vi "FPGA Digitize and Protect.vi"() -> ()   [LabVIEW 2020]
doc: "Author: Scott Hannahs <sth@magnet.fsu.edu>\nCopyright 2018 Florida State University, All rights reserved."
uses:
  SCH Test Controls/SCH Fudge Factor Array.ctl
  SCH Test Controls/SCH Fudge Factor.ctl
  SCH Test Controls/SCH Layer Error Array.ctl
  SCH Data Controls/SCH Data 2 RT.ctl
  SCH Scaling Controls/SCH Scale Factor Array.ctl
  SCH Scaling Controls/SCH Scale Factor.ctl
  SCH Data Controls/SCH Layer Voltage Array.ctl
  Init Coil Calibration/FPGA Magnet Config.ctl
  SCH Scaling Controls/SCH Joint Scale Factor Array.ctl
  SCH Scaling Controls/SCH Joint Scale Factor.ctl
  SCH Test Controls/SCH CoWound Geometric Factor.ctl
  SCH Scaling Controls/SCH CoWound Scale Factor.ctl
  SCH Data Controls/SCH Joint Voltage Array.ctl
  SCH Data Controls/SCH CoWound Volt Array.ctl
  SCH Scaling Controls/SCH SC Bus Scale Factor Array.ctl
  SCH Scaling Controls/SCH SC Bus Scale Factor.ctl
  SCH Data Controls/SCH SC Bus Volt Array.ctl
  SCH Data Controls/SCH Data 2 RT Array.ctl
  SCH Data Controls/SCH Resistive Data Array.ctl
  SCH Data Controls/SCH FXP Type.ctl
  SCH Test Controls/SCH CoWound Volt Limit.ctl
  SCH Data Controls/SCH Raw Int Data.ctl
  SCH Scaling Controls/SCH Dump Resistor Scale Factor.ctl
  SCH Data Controls/SCH Pressure Array.ctl
  SCH Data Controls/Digitizer State Enum.ctl
  SCH Data Controls/SCH Int Data with Pressure.ctl
  <vilib>/rvi/Emulation/niFpgaGetClockAttributes.vi
  <vilib>/rvi/Emulation/niFpgaSctlEmulationGetInTimedLoop.vi
  <vilib>/rvi/Emulation/niFpgaEmulationReportErrorSimple.vi
  <vilib>/rvi/Emulation/niFpgaProcessEmulError.vi
  <vilib>/rvi/eio/common/nirviEmuTemplateMethod_errors.vi
  <vilib>/rvi/Emulation/niFpgaCriticalErrorInLSC.vi
  <vilib>/rvi/Emulation/niFpgaEmulationIsFPGAContextNoSignature.vi
  <vilib>/rvi/errors/niFpgaSetErrorForExecOnDevCompSimple.vi
  <vilib>/rvi/eio/common/nirviEmuReportErrorAndStop.vi
  <vilib>/rvi/DataTransferAndStorage/Container/Common/niFpgaContainerGetUniqueNameForEmu.vi
  <vilib>/rvi/FIFO/Fifo_Resource/nirvififoEmulationSetSize.vi
  <vilib>/rvi/FIFO/Fifo_Resource/nirviFifoEmulationQueueMgr.vi
  <instcachedir>/0/nirviFifoEmulationQueueMgr_E5CAEC123FF24DC58D834DCA3CDAA9B5.lvgen/nirviFifoEmulationQueueMgr_E5CAEC123FF24DC58D834DCA3CDAA9B5_006.vi
  <vilib>/Utility/error.llb/Clear Errors.vi
  <vilib>/rvi/FIFO/Fifo_Resource/nirvififoEmulationCreateLock.vi
  <vilib>/rvi/FIFO/Fifo_Resource/nirvififoEmulationObtainLock.vi
  <vilib>/rvi/FIFO/Fifo_Resource/nirvififoEmulationReleaseLock.vi
  <vilib>/rvi/occurrence/nirviWaitOnOccurrenceBase.vi
  <vilib>/rvi/errors/nirviReportUnexpectedCaseInternalError.vi
  <vilib>/rvi/errors/nirviReportUnexpectedCaseInternalError (U32).vi
  <instcachedir>/0/nirviFifoEmulationQueueMgr_E5CAEC123FF24DC58D834DCA3CDAA9B5.lvgen/nirviFifoEmulationQueueMgr_E5CAEC123FF24DC58D834DCA3CDAA9B5_010.vi
  <vilib>/rvi/FIFO/Fifo_Resource/nirvififoEmulationDetermineInputValidOut.vi
  <instcachedir>/0/nirviFifoEmulationQueueMgr_E5CAEC123FF24DC58D834DCA3CDAA9B5.lvgen/nirviFifoEmulationQueueMgr_E5CAEC123FF24DC58D834DCA3CDAA9B5_004.vi
  <instcachedir>/0/nirviFifoEmulationQueueMgr_E5CAEC123FF24DC58D834DCA3CDAA9B5.lvgen/nirviFifoEmulationQueueMgr_E5CAEC123FF24DC58D834DCA3CDAA9B5_005.vi
  <instcachedir>/0/nirviFifoEmulationQueueMgr_E5CAEC123FF24DC58D834DCA3CDAA9B5.lvgen/nirviFifoEmulationQueueMgr_E5CAEC123FF24DC58D834DCA3CDAA9B5_007.vi
  <instcachedir>/0/nirviFifoEmulationQueueMgr_E5CAEC123FF24DC58D834DCA3CDAA9B5.lvgen/nirviFifoEmulationQueueMgr_E5CAEC123FF24DC58D834DCA3CDAA9B5_008.vi
  <instcachedir>/0/nirviFifoEmulationQueueMgr_E5CAEC123FF24DC58D834DCA3CDAA9B5.lvgen/nirviFifoEmulationQueueMgr_E5CAEC123FF24DC58D834DCA3CDAA9B5_009.vi
  <vilib>/rvi/Memory/Memory_Emulation/nirvimemoryFastEmulation.vi
  <vilib>/rvi/Memory/Memory_Emulation/nirvimemoryEmulation.vi
  <vilib>/eio/EIONode/EIONode.xnode
  <vilib>/rvi/DataTransferAndStorage/Container/XNode/niFpgaContainer.xnode
  <vilib>/rvi/FIFO/Fifo_Resource/nirvififoEmulationRead.vi
  <vilib>/rvi/FIFO/Fifo_Resource/nirvififoEmulationWrite.vi
  <vilib>/rvi/FXPMathLib/FxpInterpret/XNode/nifxpmath_Interpret.xnode
panel:
  in  "All Breaker Tick Limit":u32=400000000
  out "All Breakers Fault":bool
  in  "SCHMPS#2 Breaker Enable":bool
  out "Low Current Mode":bool
  out "Build":u8=110
  out "Fix":u8
  out "Minor":u8=6
  out "Major":u8=2
  in  "Signal Injection On":bool
  out "DAQ Zero Fault":bool
  out "SC Bus Index":i32
  out "Pressure Check Index":i32
  out "Layer Index":i32
  out "Co-Wound Index":i32
  out "Joint Index":i32
  out "Read Error Index":i32
  out "Calibrate Loop Index":i32
  out "Resistive Index":i32
  out "PS Enable Index":i32
  out "Watch Dog Index":i32
  out "Pressure Loop WDT":bool
  in  "Reset PS Enable":bool
  in  "Reset Breaker":bool
  out "Digitizer Read OK":bool
  in  "Input Select":T1(ring)
  out "uSec/Cycle":u32
  out "PS Enable":bool
  out "PS Enable Loop WDT":bool
  out "Breaker Enable":bool
  out "Resistive Loop WDT":bool
  in  "Inject Channel":i32=1
  in  "Inject Offset":fxp<+/-,16,5> format="%.3g"
  in  "Inject frequency (Hz)":fxp<+,32,16>
  out "SC Bus Loop WDT":bool
  in  "Tab Control":T2(tab)
  in  "Fudge Factors":T3=[0.048662399873137474, 0.049115100875496864, -0.0418637003749609, -0.014916900545358658, 0.07261339947581291, -0.04519769921898842, -0.00321120023727417, -0.02349269948899746, -0.0025009997189044952, 0.028547899797558784, -0.02704860083758831, 0.003521999344229698, 0.0059306006878614426, -0.00880029983818531, -0.02976590022444725, 0.03902189992368221] format="%.7g"
  in  "Layer Scale Factors":T5=[4.000479996204376, 3.5011550039052963, 3.5012779980897903, 3.5011550039052963, 3.001561000943184, 3.001561000943184, 3.5000530034303665, 3.500664994120598, 3.5011550039052963, 4.000159993767738, 3.999679997563362, 4.000159993767738, 3.998879998922348, 3.999520003795624, 3.999679997563362, 4.000320002436638, 4.000960007309914, 4.000640004873276]
  out "Error Voltages":T7 format="%.7f"
  out "Layer Voltages":T9 format="%.7f"
  out "VT Error Array":bool[](array[boolean])
  out "CoWound Volt Array":T10 format="%.4f"
  in  "Co-Wound Scale Factor":T11=60.04379999637604
  in  "Co-Wound Asymmetry Factor":T12=-0.0026702880859375 format="%.8g"
  out "Dump Resistor Voltage":T8 format="%.3f"
  in  "Dump Resistor Scale Factor":T13=204.79399999976158
  out "Joint Voltages":T14 format="%_6e"
  in  "Joint Scale Factors":T15=[0.00020059943199157715, 0.0002005249261856079, 0.00020040571689605713, 0.00020048022270202637, 0.00020040571689605713, 0.00020076334476470947, 0.00020068883895874023, 0.00020043551921844482]
  out "Joint Err Array":bool[](array[boolean])
  in  "HTS Resistance (nOhm)":T8[](array[typedef])=[0.0, 0.0] format="%_6g"
  out "RT Bus Err Array":bool[](array[boolean])
  out "HTS Bus Err Array":bool[](array[boolean])
  out "HTS Lead Warn Err Array":bool[](array[boolean])
  out "HTS Lead FRZ Err Array":bool[](array[boolean])
  out "SC Bus Volt Array":T17 format="%.8f"
  in  "SC Bus Scale":T18=[0.10001799464225769, 0.10001499950885773, 0.0009999573230743408, 0.0009999573230743408, 0.0002005249261856079, 0.0002006441354751587]
  out "SC Bus Err Array":bool[](array[boolean])
  in  "HTS Offset (microV)":T8[](array[typedef])=[0.0, 0.0] format="%_6g"
  out "Dump File Enable":bool
  out "I*Temp Fault":bool
  out "Coil Volt Fault":bool
  out "Current Fault":bool
  out "Pressure Fault":bool
  out "Resistive Data":T20 format="%.4g"
  in  "Magnet Configuration Data":T21={"#Coils"=4, "Coil Inductances"=[0.10000002384185791, 0.3999999761581421, 0.6000000238418579, 1.199999988079071], "Max Coil Currents"=[19.899999976158142, 19.899999976158142, 19.899999976158142, 19.899999976158142], "Max Coil Volt Dev"=[1.800000011920929, 2.100000023841858, 3.100000023841858, 2.600000023841858], "Coil A Coefficients"=[0.8209999799728394, 0.00010001659393310547, 5.960464477539063e-08], "Coil B Coefficients"=[0.8999999761581421, 0.00019997358322143555, 2.9802322387695312e-06], "Coil C Coefficients"=[1.100000023841858, 0.0, 0.0], "Coil D Coefficients"=[1.0, 0.0009999871253967285, 0.0], "Max Coil Temp"=[100.0, 80.0, 80.0, 60.0], " Pressure Range"=[29.30000001192093, 32.30000001192093], "Temp Coef"=[0.0031999945640563965, 0.0031999945640563965, 0.0029000043869018555, 0.004100024700164795], "Offsets"=[0.0, 0.0, -5.0, -5.0, 0.0, 0.0, 0.0, 0.0, 0.0, 0.0, 0.0, 0.0, 0.0, 0.0, 0.0], "Scale Factors"=[20.0, 20.0, 4.2670000195503235, 4.269999980926514, 2.0, 1.0, 1.0, 1.0, 1.0, 1.0, -2.0, 30.08600002527237, 29.861999988555908, 35.50199997425079, 35.56999999284744]} {"Coil D Coefficients" format="%_6g"; "Coil C Coefficients" format="%_6g"; "Coil B Coefficients" format="%_6g"; "Scale Factors" format="%_5g"; "Offsets" format="%_5g"; "Temp Coef" format="%_6g"; "Max Coil Temp" format="%_6g"; "Max Coil Volt Dev" format="%_6g"; "Max Coil Currents" format="%_6g"; "Coil Inductances" format="%_6g"; "Pressure Range" format="%_6g"; "Coil A Coefficients" format="%_6g"}
  out "dI/dt":fxp<+/-,34,10>
  out "Temp Faults":bool[](array[boolean])
  out "Coil V Faults":bool[](array[boolean])
  out "Bore Tube Fault":bool
  out "Active":bool
  out "Coil Ref Voltages":T8[](array[typedef]) format="%_6g"
  in  "Cooldown Mode":bool
  in  "Pressure Scale Factor":T8[](array[typedef])=[1.723690003156662, 1.723690003156662, 1.723690003156662, 1.723690003156662] format="%_6g"
  out "Pressures":T22 format="%.3g"
  out "Pressure Limit Err Array":bool[](array[boolean])
  out "Offset":T23
  out "Calibrate Index":i16
  out "Scale":T23
  in  "Pressure Outlet Cooldown Limit":T24=10.0 format="%.5g"
  in  "Pressure Inlet Cooldown Limit":T24=12.0 format="%.5g"
  in  "Delay Ticks Between Bkr Reset":u32=1200000000
  in  "Sync Guard Data":fxp<+/-,38,12>[](array[numeric])=[888.2284999489784, 399.7682446986437, -617.0920498371124] format="%.9g"
  in  "Low Current Delay Factor":u16=100
  in  "Low Current Ticks":u32=400000000
  in  "Low Current (kA)":T8=0.04500000178813934 format="%_6g"
  in  "Digitize # Bits":u32=16
  in  "Digitize Read Delay Ticks":u32=13
  in  "Convert Clock Ticks":u32=20
  in  "Digitize Reset Ticks":u32=400
  in  "HTS Lead Warn":T8=0.0010000020265579224 format="%_6g"
  in  "HTS Lead FRZ":T8=0.006999999284744263 format="%_6g"
  in  "Res Lead Tick Limit":u32=4000000
  in  "Res Lead Limit":T8=0.001953125 format="%_6g"
  in  "HTS Lead Tick Limit":u32=4000000
  in  "HTS Lead Trip":T8=0.20000000298023224 format="%_6g"
  in  "Activation Current (kA)":T8=0.5 format="%_6g"
  in  "Pressure Outlet Limit (BarA)":T24=5.0 format="%.5g"
  in  "Bore Tube Volt Limit":T8=0.5999999940395355 format="%_6g"
  in  "Pressure Inlet Limit (BarA)":T24=6.0 format="%.5g"
  in  "dI/dT scaling":fxp<+/-,35,11>=38.14697265625 caption="Inverse Seconds,\n40,000,000/(4096 * 256)" format="%.11g"
  in  "Res Mag dI/dt Delay":u32=256
  in  "DAQ Cycle Ticks":u32=4096
  in  "ResMag Tick Limit":u32=1000000
  in  "SC Bus Tick Limit":u32=4000000
  in  "SC Bus Limit":T8=0.001953125 format="%_6g"
  in  "CoWound Tick Limit":u32=4000000
  in  "CoWound Volt Limit":T25=0.20001220703125
  in  "Joint Volt Limit":T8=9.98377799987793e-07 format="%_6g"
  in  "Joint Tick Limit":u32=4000000
  in  "VT Quench Volt Limit":T24=0.1999969482421875 format="%.5g"
  in  "VT Quench Tick Limit":u32=4000000
  out "Data Size":i32
  in  "Ln2 Filter Size":i16=10
  out "Chassis Temperature":fxp<+/-,16,14> format="%.2f"
  in  "# Consecutive Zeros Fault":i16=1000
  in  "Digitize Convert Ticks":u32=200
  in  "Ticks to Close Relief":u32=80000000
  in  "Breaker Reset Ticks":u32=40000000 caption="Tick Count(Ticks)"
  in  "PS Enable Reset Ticks":u32=40000000 caption="Tick Count(Ticks)"
  in  "Reset Digitizer Ticks":u32=40000000 caption="Tick Count(Ticks)"
  in  "Breaker 6":bool
  in  "Breaker 5":bool
  in  "Breaker 4":bool
  in  "Breaker 3":bool
  in  "Breaker 2":bool
  in  "Breaker 1":bool
  out "Breaker Neg 6 Closed":bool
  out "Breaker Neg 5 Closed":bool
  out "Breaker Neg 4 Closed":bool
  out "Breaker Pos 3 Closed":bool
  out "Breaker Pos 2 Closed":bool
  out "Breaker Pos 1 Closed":bool
  out "Pwr 125V Err":bool
  out "Pwr 24V Aux Err":bool
  out "Pwr 24V Pri Err":bool
  out "Pwr 5V Aux Err":bool
  out "Pwr 5V Pri Err":bool
  out "Pwr ±15V Aux Err":bool
  out "Pwr ±15V Pri Err":bool
  out "Proto VT Quench":bool
  out "VT Quench Err":bool
  out "Overall WDT":bool
  out "Joint Limit Err":bool
  out "Proto Joint Volt":bool
  out "Proto Co-Wournd Limit":bool
  out "Co-Wound Limit Err":bool
  out "Proto SC Bus Limit":bool
  out "SC Bus Limit Err":bool
  out "Proto ResMag Limit":bool
  out "ResMag Limit Err":bool
  out "Layer Loop WDT OK":bool
  out "DAQ Loop WDT OK":bool
  out "Joint Loop WDT OK":bool
  out "Co-Wound Loop WDT OK":bool
  out "SC Bus Loop WDT OK":bool
  out "Resistive Loop WDT OK":bool
  out "PS Enable Loop WDT OK":bool
  out "Pressure Loop WDT OK":bool
  out "Pressure Limit Err":bool
  out "Breaker First Error":u64 format="%010x"
  out "PS Enable First Error":u32 format="%07x"
  out "HTS Bus Limit Err":bool
  out "RT Bus Limit Err":bool
  out "Proto HTS Bus Limit":bool
  out "Proto RT Bus Limit":bool
  out "Timed Out? Calc Read":bool
  out "Timed Out? FIFO Raw":bool
  out "Timed Out? FIFO2RT Filter":bool
  out "Timed Out? Joint Read":bool
  out "Timed Out? Co-Wound Read":bool
  out "Timed Out? SC Bus Read":bool
  out "Timed Out? ResMag Read":bool
  out "Timed Out? FIFO2RT Raw":bool
  out "DAQ Zero Fault Channel":bool[](array[boolean])
  out "All Breakers Closed":bool
  out "Raw Data":T26=[0.0, 0.0, 0.0, 0.0, 0.0, 0.0, 0.0, 0.0, 0.0, 0.0, 0.0, 0.0, 0.0, 0.0, 0.0, 0.0, 0.0, 0.0, 0.0, 0.0, 0.0, 0.0, 0.0, 0.0, 0.0, 0.0, 0.0, 0.0, 0.0, 0.0, 0.0, 0.9999999701976776, 0.0, 0.0, -1.0, 0.9999999701976776, -1.0, -1.0, 0.9971923828125, 0.0, 0.0, 0.0, 0.0, 0.0, 0.0, -1.0, 0.0, 0.0, 0.0, 0.0, 0.0, 0.0, 0.0, 0.0] format="%_6g"
  out "Filt Data":T26=[0.0, 0.0, 0.0, 0.0, 0.0, 0.0, 0.0, 0.0, 0.0, 0.0, 0.0, 0.0, 0.0, 0.0, 0.0, 0.0, 0.0, 0.0, 0.0, 0.0, 0.0, 0.0, 0.0, 0.0, 0.0, 0.0, 0.0, 0.0, 0.0, 0.0, 0.0, 0.9999999701976776, 0.0, 0.0, -1.0, 0.9999999701976776, -1.0, -1.0, 0.9971923828125, 0.0, 0.0, 0.0, 0.0, 0.0, 0.0, -1.0, 0.0, 0.0, 0.0, 0.0, 0.0, 0.0, 0.0, 0.0] format="%_6g"
  in  "Stop WD Loop":bool
  out "16 Bigitizer output":T23 format="%.0x"
  out "Co-Wound Loop WDT":bool
  out "Joint Loop WDT":bool
  out "DAQ Loop WDT":bool
  out "Layer Loop WDT":bool
  in  "Reset Digitizers":bool
  in  "stop":bool
  out "Main Index":i32
  # "SCH Protection FPGA System"
  # "."
  # "."
  # "."
  # "Sum of Layers"
  # "Co-Wound Voltage"
  # "`"
  # "Cold Mass Inlet Joint\nCold Mass Outlet Joint\nInlet Lead 4K Joint\nOutlet Lead 4K Joint\nHF-MF Joint\nMF-LF1 Joint\nLF1-LF2 Joint\nLF2-LF3 Joint"
  # "Inlet RT to 77K\nOutlet RT to 77K\nInlet 77K to 4K\nOutlet 77K to 4K\nInlet SC Bus\nOutlet SC Bus"
  # "Resistive Inlet Temperature\nResistive Outlet Temperature\nResistive Inlet Pressure\nResistive Outlet Pressure\nCurrent (kA)\nWatchdog Timer Input\nPower Supply Enable\nBreaker Enable\nCell Fault\nWatchdog Timer Fault\nBore Tube Voltage\nResistive Coil A Voltage\nResistive Coil B Voltage\nResistive Coil C Voltage\nResistive Coil D Voltage"
  # "mH"
  # "kA"
  # "V"
  # "mOhm"
  # "mOhm"
  # "mOhm"
  # "mOhm"
  # "Deg C"
  # "bar"
  # "1/Deg C"
  # "Tin"
  # "Tout"
  # "Pin"
  # "Pout"
  # "I"
  # "WDTin"
  # "PSEnb"
  # "BrkrEnb"
  # "CellFLT"
  # "WDT Trip"
  # "BTvolt"
  # "Va"
  # "Vb"
  # "Vc"
  # "Vd"
  # "Tin"
  # "Tout"
  # "Pin"
  # "Pout"
  # "I"
  # "WDTin"
  # "PSEnb"
  # "BrkrEnb"
  # "CellFLT"
  # "WDT Trip"
  # "BTvolt"
  # "Va"
  # "Vb"
  # "Vc"
  # "Vd"
  # "PI751 Inlet\nPI752 Inlet\nPI753 Inlet\nPI755 Outlet"
  # "SCH Protection Globals"
  # "All Clock Ticks are at 40 MHz"
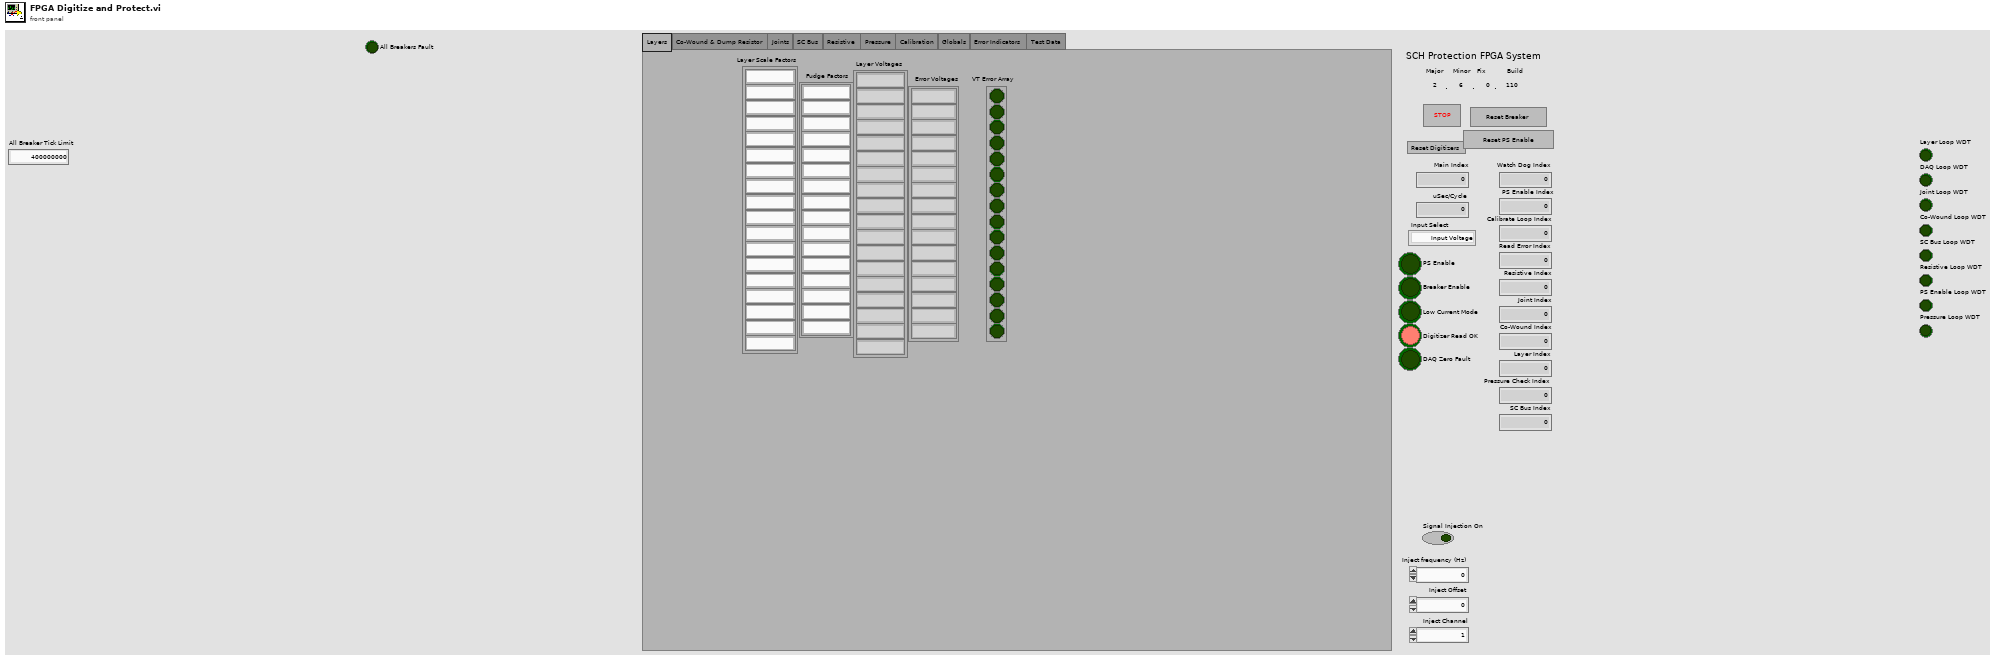
[diagram p1: front panel]
types:
  T1 = enum16{"Input Voltage", "Zero Voltage", "Calibrate Voltage"}
  T2 = enum32{"Layers", "Co-Wound & Dump Resistor", "Joints", "SC Bus", "Resistive", "Pressure", "Calibration", "Globals", "Error Indicators", "Test Data"}
  T3 = typedef "SCH Fudge Factor Array.ctl" = T4[]
  T4 = typedef "SCH Fudge Factor.ctl" = fxp<+/-,32,3>
  T5 = typedef "SCH Scale Factor Array.ctl" = T6[]
  T6 = typedef "SCH Scale Factor.ctl" = fxp<+/-,38,12>
  T7 = typedef "SCH Layer Error Array.ctl" = T8[]
  T8 = typedef "SCH Data 2 RT.ctl" = fxp<+/-,38,12>
  T9 = typedef "SCH Layer Voltage Array.ctl" = T8[]
  T10 = typedef "SCH CoWound Volt Array.ctl" = T8[]
  T11 = typedef "SCH CoWound Scale Factor.ctl" = fxp<+/-,38,12>
  T12 = typedef "SCH CoWound Geometric Factor.ctl" = fxp<+/-,16,0>
  T13 = typedef "SCH Dump Resistor Scale Factor.ctl" = fxp<+/-,38,12>
  T14 = typedef "SCH Joint Voltage Array.ctl" = T8[]
  T15 = typedef "SCH Joint Scale Factor Array.ctl" = T16[]
  T16 = typedef "SCH Joint Scale Factor.ctl" = fxp<+/-,38,12>
  T17 = typedef "SCH SC Bus Volt Array.ctl" = T8[]
  T18 = typedef "SCH SC Bus Scale Factor Array.ctl" = T19[]
  T19 = typedef "SCH SC Bus Scale Factor.ctl" = fxp<+/-,38,12>
  T20 = typedef "SCH Resistive Data Array.ctl" = T8[]
  T21 = typedef "FPGA Magnet Config.ctl" = cluster{"#Coils":u32, "Coil Inductances":T8[], "Max Coil Currents":T8[], "Max Coil Volt Dev":T8[], "Coil A Coefficients":T8[], "Coil B Coefficients":T8[], "Coil C Coefficients":T8[], "Coil D Coefficients":T8[], "Max Coil Temp":T8[], " Pressure Range":T8[], "Temp Coef":T8[], "Offsets":T8[], "Scale Factors":T8[]}
  T22 = typedef "SCH Pressure Array.ctl" = T8[]
  T23 = typedef "SCH Raw Int Data.ctl" = i16[]
  T24 = typedef "SCH FXP Type.ctl" = fxp<+/-,38,12>
  T25 = typedef "SCH CoWound Volt Limit.ctl" = fxp<+/-,16,1>
  T26 = typedef "SCH Data 2 RT Array.ctl" = T8[]
  T27 = typedef "Digitizer State Enum.ctl" = enum16{"Reset", "StartCnvt"}
  T28 = typedef "SCH Int Data with Pressure.ctl" = fxp<+/-,19,5>[]
  T29 = typedef "SCH All FXP Data.ctl" = fxp<+/-,19,5>[]
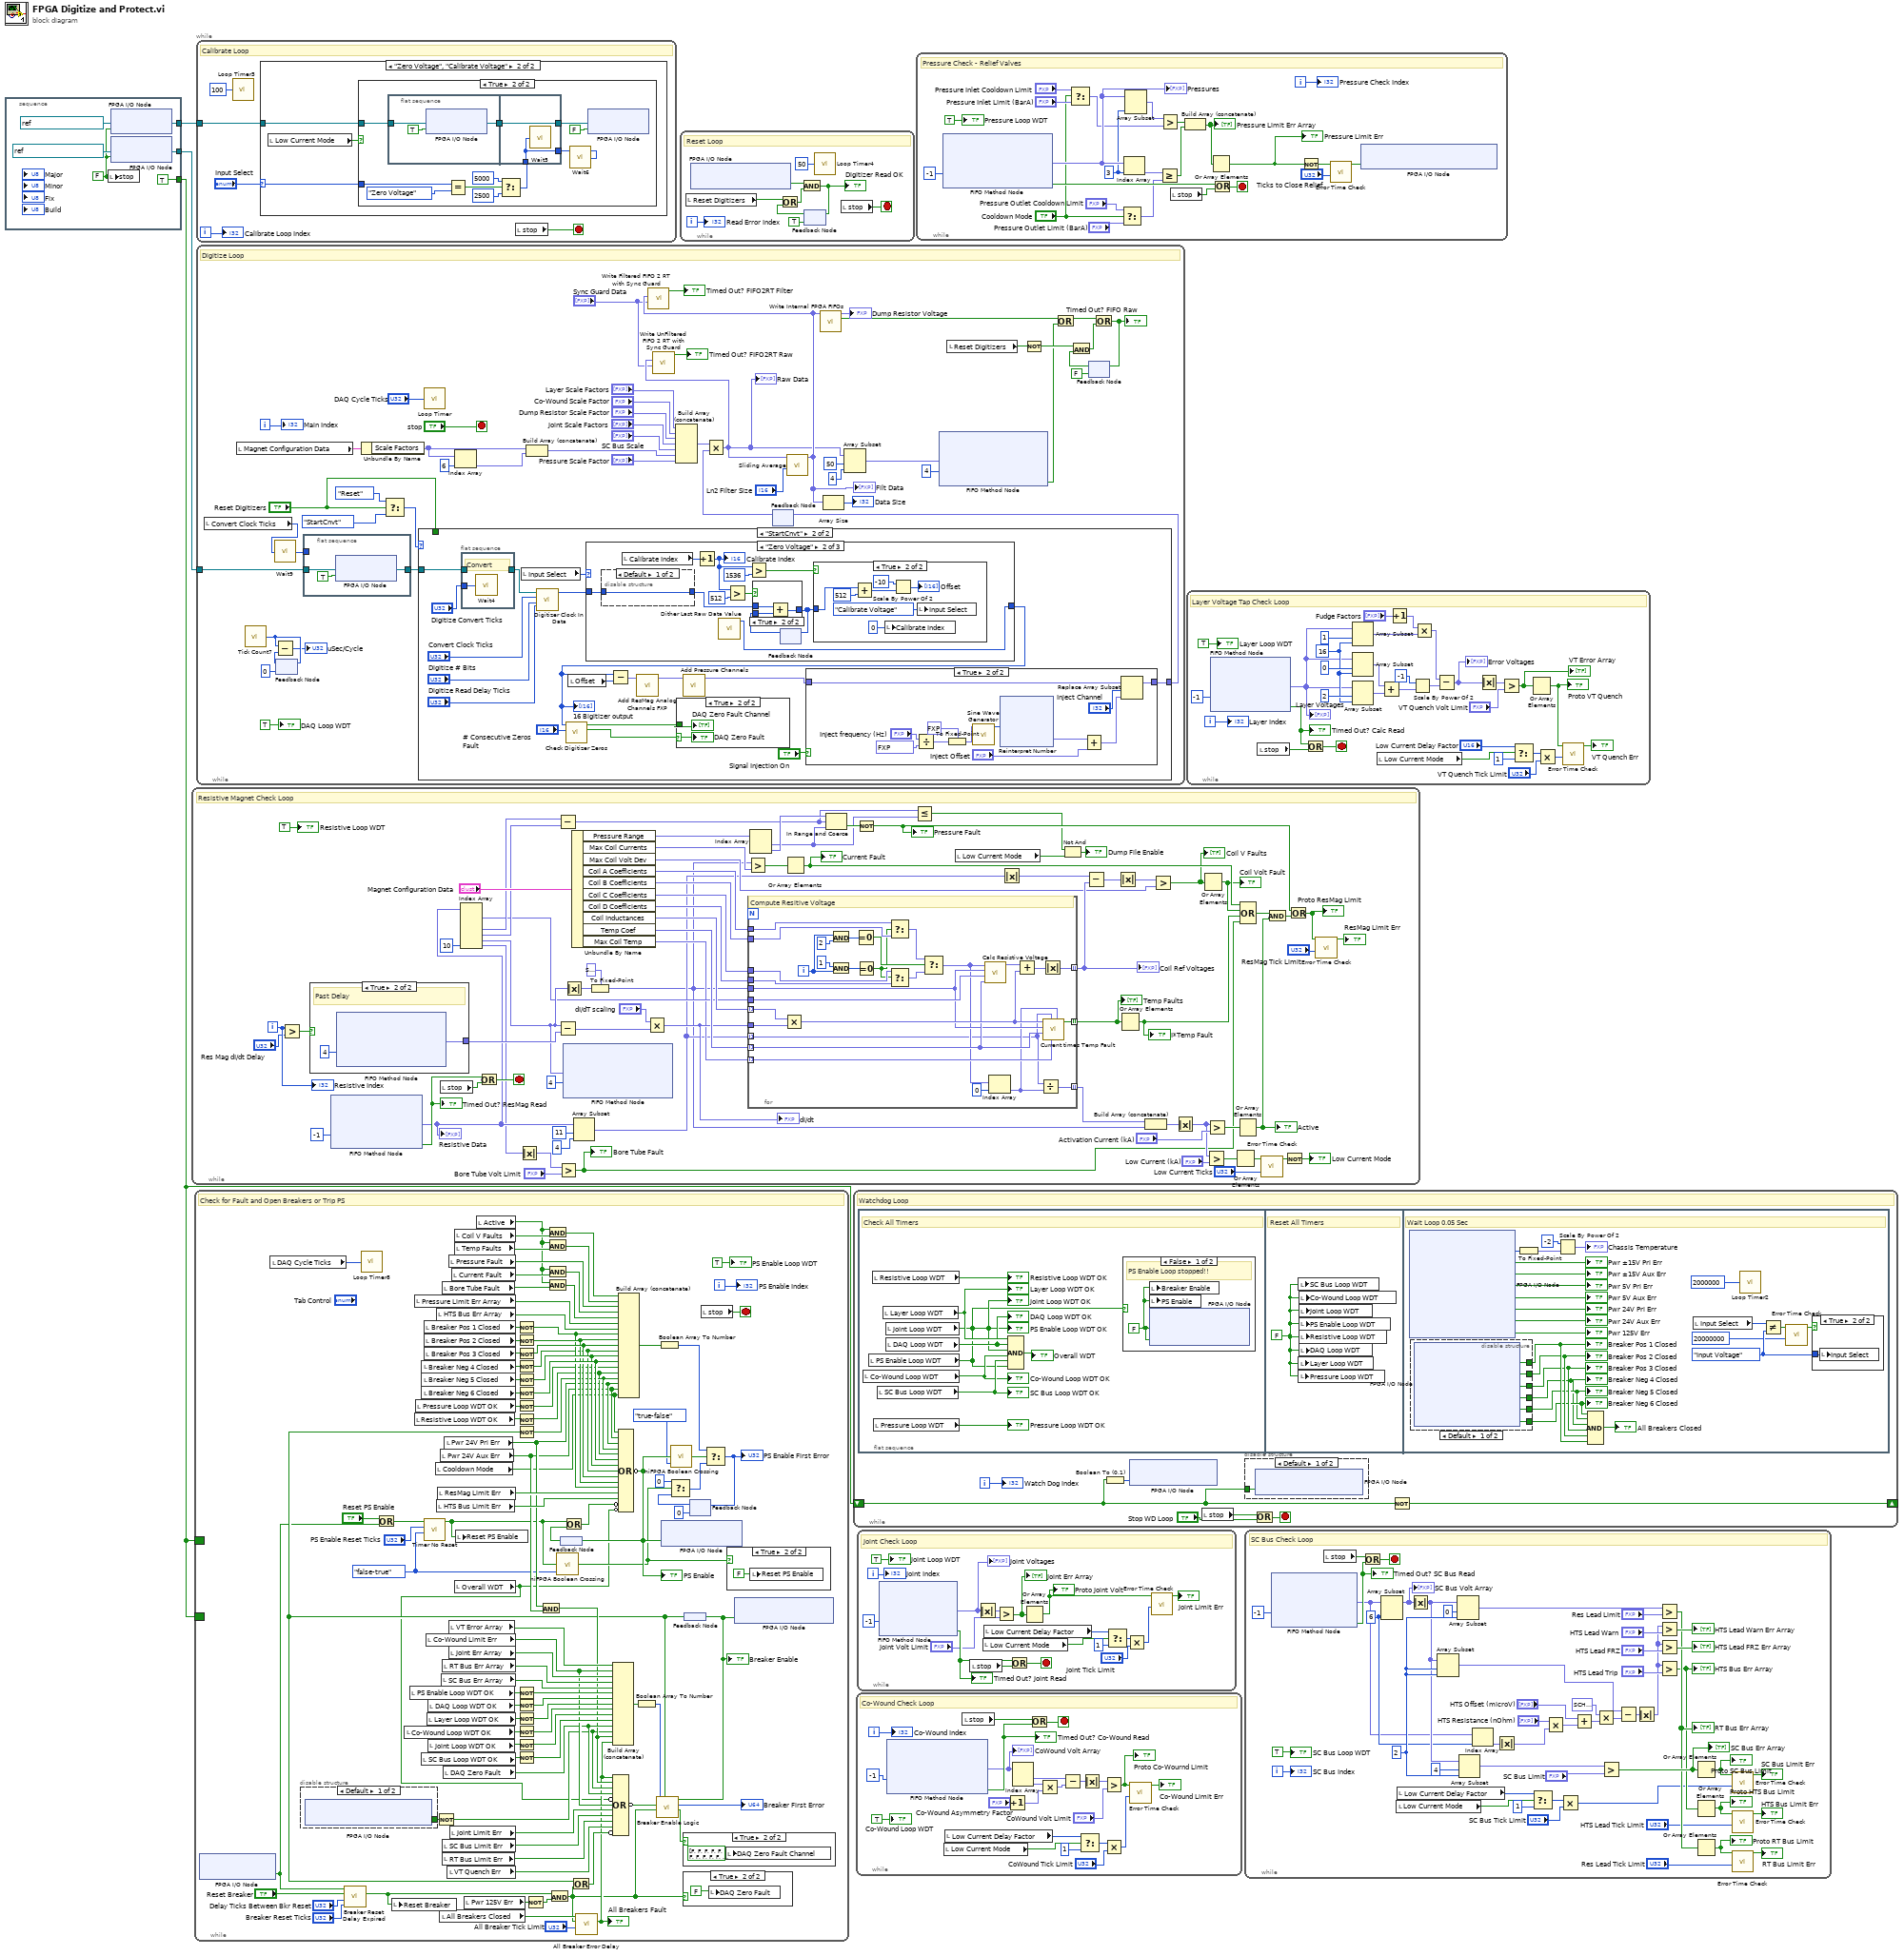
[diagram p0: block diagram]
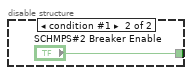
[diagram p2: hidden frame]
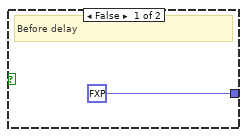
[diagram p6: hidden frame]
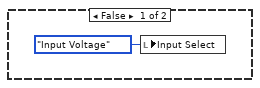
[diagram p8: hidden frame]
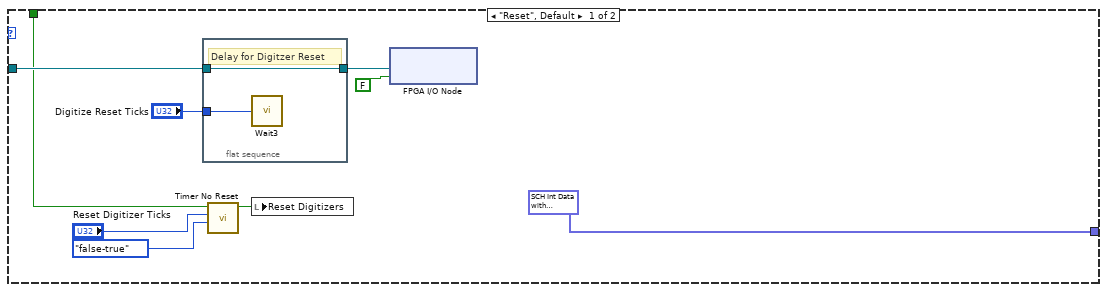
[diagram p9: hidden frame]
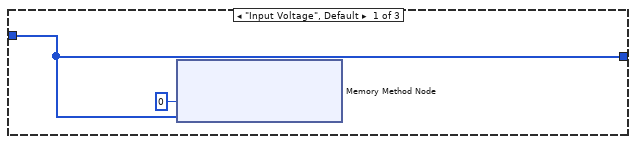
[diagram p12: hidden frame]
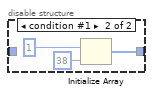
[diagram p13: hidden frame]
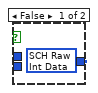
[diagram p15: hidden frame]
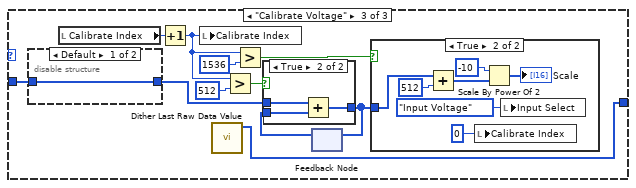
[diagram p16: hidden frame]
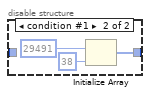
[diagram p17: hidden frame]
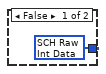
[diagram p19: hidden frame]
diagram:
  n1 = stacked-sequence {
    tunnel: [w9] -> w3
    tunnel: [TRUE] -> w1
    tunnel: [w4] -> w2
    frame #0 {
      w5 = FALSE ("Connector0/DIO0")
      n2 = local write "stop"(w5) -> ()
      n3 = xnode "FPGA I/O Node"("I/O Item"=w5, "FPGA I/O In"=refnum<k21> "Digitizer Calibrate") -> ("FPGA I/O Out"=w4:refnum<k21>)
      n4 = xnode "FPGA I/O Node"("I/O Item"=w5, "FPGA I/O In"=refnum<k21> "Digitizer Clock Data") -> ("FPGA I/O Out"=w9:refnum<k21>)
    }
  }
  n5 = while {
    i -> [w55]
    stop <- w83 stop-if-true
    # "Resistive Magnet Check Loop"
    n6 = Greater?(x=w55, y="Res Mag dI/dt Delay") -> (0:w54:bool)
    n7 = case shown="True" w54 {
      tunnel: [fxp<+/-,26,10> 0.0 ("Element") w116] -> w57
      frame False {
        # "Before delay"
      }
      frame True {
        # "Past Delay"
        n8 = xnode ("FIFO Method Node")("Timeout"=4) -> ("Element"=w116:fxp<+/-,26,10>)  [unwired: 1 in, 2 out]
      }
    }
    n9 = xnode ("FIFO Method Node")("Timeout"=-1) -> ("Element"=w41:fxp<+/-,38,12>[], "Timed Out?"=w76:bool)  [unwired: 1 in, 1 out]
    "Timed Out? ResMag Read" <- w76
    "Resistive Data" <- w41
    n10 = local read "stop"() -> (w82:bool)
    n11 = Index Array(array=w41, index #6=10 ("index")) -> (element #1=w49:fxp<+/-,38,12>, element #3=w79:fxp<+/-,38,12>, element #4=w78:fxp<+/-,38,12>, element #5=w53:fxp<+/-,38,12>, element #6=w39:fxp<+/-,38,12>)  [unwired: 5 in, 1 out]
    n12 = Or(x=w76, y=w82) -> (x .or. y?=w83:bool)
    n13 = Absolute Value(x=w39) -> (abs(x)=w43:fxp<+,38,12>)
    n14 = Subtract(x=w79, y=w78) -> (x-y=w26:fxp<+/-,38,12>)
    n15 = Subtract(x=w53, y=w57) -> (x-y=w51:fxp<+/-,39,13>)
    n16 = Greater?(x=w43, y="Bore Tube Volt Limit") -> (0:w10:bool)
    "Bore Tube Fault" <- w10
    n17 = Absolute Value(x=w53) -> (abs(x)=w34:fxp<+,38,12>)
    n18 = xnode ("FIFO Method Node")("Element"=w53, "Timeout"=4) -> ()  [unwired: 1 in, 2 out]
    n19 = Unbundle By Name("Magnet Configuration Data") -> ("Pressure Range"=w80:T8[], "Max Coil Currents"=w73:T8[], "Max Coil Volt Dev"=w65:T8[], "Coil A Coefficients"=w59:T8[], "Coil B Coefficients"=w62:T8[], "Coil C Coefficients"=w61:T8[], "Coil D Coefficients"=w60:T8[], "Coil Inductances"=w52:T8[], "Temp Coef"=w50:T8[], "Max Coil Temp"=w47:T8[])
    n20 = Array Subset(array=w41, index=11, length=4) -> (w30:fxp<+/-,38,12>[])
    n21 = To Fixed-Point(fixed-point type=T8 0.0, number=w34) -> (fixed-point=w22:T8)
    n22 = Multiply(x="dI/dT scaling", y=w51) -> (x*y=w48:fxp<+/-,34,10>)
    "dI/dt" <- w48
    n23 = Greater?(x=w22, y=w73) -> (0:w72:bool[])
    n24 = for {
      tunnel: w22 -> [w104]
      tunnel: [w88] -> w70 mode=indexing
      tunnel: w59 -> [w95]
      tunnel: w62 -> [w94]
      tunnel: w61 -> [w93]
      tunnel: w60 -> [w92]
      tunnel: w52 -> [w111] mode=indexing
      tunnel: w48 -> [w110]
      tunnel: w50 -> [w107] mode=indexing
      tunnel: w49 -> [w109]
      tunnel: w30 -> [w85] mode=indexing
      tunnel: [w106] -> w46 mode=indexing
      tunnel: w47 -> [w105] mode=indexing
      tunnel: [w86] -> w35 mode=indexing
      i -> [w96]
      # "Compute Resitive Voltage"
      n25 = Multiply(x=w111, y=w110) -> (x*y=w108:T8)
      n26 = And(x=w96, y=2) -> (x .and. y?=w100:i32)
      n27 = And(x=1, y=w96) -> (x .and. y?=w101:i32)
      n28 = Equal To 0?(x=w100) -> (x = 0?=w99:bool)
      n29 = Equal To 0?(x=w101) -> (x = 0?=w91:bool)
      n30 = Select(t=w95, s=w91, f=w94) -> (s? t:f=w97:T8[])
      n31 = Select(t=w93, s=w91, f=w92) -> (s? t:f=w98:T8[])
      n32 = Select(t=w97, s=w99, f=w98) -> (s? t:f=w90:T8[])
      n33 = call "Calc Resistive Voltage.vi"("Alpha"=w107, "T inlet"=w109, "Current"=w104, "Coil Coefficients"=w90) -> ("Voltage"=w113:T8)  [unwired: 6 in, 1 out]
      n34 = Index Array(array=w90, index=0) -> (element=w87:T8)
      n35 = Add(x=w113, y=w108) -> (x+y=w112:T8)
      n36 = Divide(x=w85, y=w87) -> (x/y=w86:T8)
      n37 = Absolute Value(x=w112) -> (abs(x)=w88:fxp<+,38,12>)
      n38 = call "Current times Temp Fault.vi"("Resistance"=w87, "Max Temp"=w105, "Coil Voltage"=w85, "Temp Coef"=w107, "Current"=w104, "Inductive V"=w108) -> ("I * Temp Fault"=w106:bool)  [unwired: 5 in]
    }
    "Temp Faults" <- w46
    "Coil Ref Voltages" <- w70
    n39 = Index Array(array=w80) -> (element #1=w27:T8, element #2=w75:T8)  [unwired: 2 in]
    n40 = Or Array Elements(Boolean array=w72) -> (logical OR=w67:bool)
    "Current Fault" <- w67
    n41 = In Range and Coerce(upper limit=w75, x=w26, lower limit=w27) -> (In Range?=w74:bool)  [unwired: 1 out]
    n42 = Not(x=w74) -> (.not. x?=w29:bool)
    "Pressure Fault" <- w29
    n43 = Less Or Equal?(x=w26, y=w27) -> (x <= y?=w25:bool)
    n44 = local read "Low Current Mode"() -> (w13:bool)
    n45 = Absolute Value(x=w30) -> (abs(x)=w24:fxp<+,38,12>[])
    n46 = Not And(1:w13, 2:w25) -> (0:→"Dump File Enable":bool)
    n47 = Subtract(x=w24, y=w70) -> (x-y=w68:fxp<+/-,34,10>[])
    n48 = Absolute Value(x=w68) -> (abs(x)=w66:fxp<+,34,10>[])
    n49 = Or Array Elements(Boolean array=w46) -> (logical OR=w23:bool)
    "I*Temp Fault" <- w23
    n50 = Build Array (concatenate)(w35, w22) -> (w32:T8[])
    n51 = Greater?(x=w66, y=w65) -> (0:w64:bool[])
    "Coil V Faults" <- w64
    n52 = Absolute Value(x=w32) -> (abs(x)=w12:fxp<+,38,12>[])
    n53 = Or Array Elements(Boolean array=w64) -> (logical OR=w63:bool)
    "Coil Volt Fault" <- w63
    n54 = Greater?(x=w12, y="Low Current (kA)") -> (0:w19:bool[])
    n55 = Greater?(x=w12, y="Activation Current (kA)") -> (0:w36:bool[])
    n56 = Or Array Elements(Boolean array=w19) -> (logical OR=w11:bool)
    n57 = Or Array Elements(Boolean array=w36) -> (logical OR=w33:bool)
    "Active" <- w33
    n58 = Compound Arithmetic op=OR(w67, w63, w23, w10) -> (w71:bool)
    n59 = call "Error Time Check.vi"("Ticks Until Trigger"="Low Current Ticks", "Limit Exceeded"=w11) -> ("Limit Triggered"=w21:bool)  [unwired: 9 in]
    n60 = And(x=w71, y=w33) -> (x .and. y?=w37:bool)
    n61 = Not(x=w21) -> (.not. x?=→"Low Current Mode":bool)
    n62 = Or(x=w29, y=w37) -> (x .or. y?=w16:bool)
    "Proto ResMag Limit" <- w16
    n63 = call "Error Time Check.vi"("Ticks Until Trigger"="ResMag Tick Limit", "Limit Exceeded"=w16) -> ("Limit Triggered"=→"ResMag Limit Err":bool)  [unwired: 9 in]
    "Resistive Loop WDT" <- TRUE
    "Resistive Index" <- w55
  }
  n64 = while {
    border: w1 -> [_]
    border: w1 -> [_]
    i -> [w177]
    stop <- w217 stop-if-true
    w122 = enum8{"either", "false-true", "true-false"}."false-true" ("Direction")
    # "Check for Fault and Open Breakers or Trip PS"
    n65 = xnode "FPGA I/O Node"() -> ("Reset Switch"=w130:bool)  [unwired: 1 in, 1 out]
    n66 = local read "DAQ Cycle Ticks"() -> (w171:u32)
    n67 = disable-structure shown="Default" {
      disable-tunnel: [w218 "SCHMPS#2 Breaker Enable"] -> w145
      frame condition #0 (active) {
        n68 = xnode "FPGA I/O Node"() -> ("SCHMPS#2 Breaker Enable"=w218:bool)  [unwired: 1 in, 1 out]
      }
      frame condition #1 {
      }
    }
    n69 = call "Breaker Reset Delay Expired.vi"("Breaker Reset Ticks"="Breaker Reset Ticks", "Delay (Ticks)"="Delay Ticks Between Bkr Reset", "Reset Breaker"="Reset Breaker", "Reset Switch"=w130) -> ("Reset Breaker Out"=w118:bool)  [unwired: 6 in, 1 out]
    n70 = call "Loop Timer8"("Count(Ticks)"=w171) -> ()  [unwired: 1 out]
    n71 = Or(x="Reset PS Enable", y=w130) -> (x .or. y?=w124:bool)
    n72 = local write "Reset Breaker"(w118) -> ()
    n73 = local read "Co-Wound Loop WDT OK"() -> (w202:bool)
    n74 = local read "PS Enable Loop WDT OK"() -> (w204:bool)
    n75 = local read "Resistive Loop WDT OK"() -> (w156:bool)
    n76 = local read "Pressure Limit Err Array"() -> (w196:bool[])
    n77 = local read "Pressure Loop WDT OK"() -> (w157:bool)
    n78 = local read "SC Bus Loop WDT OK"() -> (w134:bool)
    n79 = local read "Breaker Neg 4 Closed"() -> (w165:bool)
    n80 = local read "Breaker Neg 5 Closed"() -> (w164:bool)
    n81 = local read "Breaker Neg 6 Closed"() -> (w163:bool)
    n82 = local read "Breaker Pos 1 Closed"() -> (w168:bool)
    n83 = local read "Breaker Pos 2 Closed"() -> (w167:bool)
    n84 = local read "Breaker Pos 3 Closed"() -> (w166:bool)
    n85 = call "Timer No Reset.vi"("Direction"=w122, "Tick Count(Ticks)"="PS Enable Reset Ticks", "Start Timer"=w124) -> ("Timer Running"=w120:bool)  [unwired: 8 in]
    n86 = local read "Co-Wound Limit Err"() -> (w152:bool)
    n87 = local read "Layer Loop WDT OK"() -> (w203:bool)
    n88 = local read "DAQ Loop WDT OK"() -> (w183:bool)
    n89 = local read "Joint Loop WDT OK"() -> (w201:bool)
    n90 = local read "Cooldown Mode"() -> (w117:bool)
    n91 = Not(x=w145) -> (.not. x?=w139:bool)
    n92 = local read "HTS Bus Err Array"() -> (w175:bool[])
    n93 = local read "HTS Bus Limit Err"() -> (w176:bool)
    n94 = local read "ResMag Limit Err"() -> (w211:bool)
    n95 = local read "All Breakers Closed"() -> (w129:bool)
    n96 = local read "Pwr 24V Aux Err"() -> (w146:bool)
    n97 = local read "SC Bus Err Array"() -> (w206:bool[])
    n98 = local read "Bore Tube Fault"() -> (w191:bool)
    n99 = local read "RT Bus Err Array"() -> (w173:bool[])
    n100 = local read "SC Bus Limit Err"() -> (w215:bool)
    n101 = local read "RT Bus Limit Err"() -> (w174:bool)
    n102 = local read "DAQ Zero Fault"() -> (w149:bool)
    n103 = local read "Pwr 24V Pri Err"() -> (w147:bool)
    n104 = local read "VT Quench Err"() -> (w214:bool)
    n105 = local read "Pressure Fault"() -> (w193:bool)
    n106 = local read "VT Error Array"() -> (w208:bool[])
    n107 = local read "Joint Err Array"() -> (w207:bool[])
    n108 = local read "Joint Limit Err"() -> (w216:bool)
    n109 = local read "Current Fault"() -> (w192:bool)
    n110 = local read "Coil V Faults"() -> (w195:bool[])
    n111 = local read "Temp Faults"() -> (w194:bool[])
    n112 = local read "Overall WDT"() -> (w121:bool)
    n113 = local write "Reset PS Enable"(w120) -> ()
    n114 = local read "Pwr 125V Err"() -> (w119:bool)
    n115 = local read "Active"() -> (w140:bool)
    n116 = Not(x=w168) -> (.not. x?=w158:bool)
    n117 = Not(x=w167) -> (.not. x?=w159:bool)
    n118 = Not(x=w166) -> (.not. x?=w160:bool)
    n119 = Not(x=w165) -> (.not. x?=w155:bool)
    n120 = Not(x=w164) -> (.not. x?=w161:bool)
    n121 = Not(x=w163) -> (.not. x?=w162:bool)
    n122 = Not(x=w157) -> (.not. x?=w153:bool)
    n123 = Not(x=w156) -> (.not. x?=w150:bool)
    n124 = Not(x=w204) -> (.not. x?=w184:bool)
    n125 = Not(x=w183) -> (.not. x?=w182:bool)
    n126 = Not(x=w203) -> (.not. x?=w181:bool)
    n127 = Not(x=w202) -> (.not. x?=w180:bool)
    n128 = Not(x=w201) -> (.not. x?=w179:bool)
    n129 = Not(x=w134) -> (.not. x?=w178:bool)
    n130 = Not(x=w119) -> (.not. x?=w138:bool)
    n131 = And(x=w147, y=w146) -> (x .and. y?=w148:bool)
    n132 = And(x=w140, y=w195) -> (x .and. y?=w144:bool[])
    n133 = And(x=w140, y=w194) -> (x .and. y?=w143:bool[])
    n134 = And(x=w140, y=w192) -> (x .and. y?=w142:bool)
    n135 = And(x=w140, y=w191) -> (x .and. y?=w141:bool)
    n136 = And(x=w118, y=w138) -> (x .and. y?=w126:bool)
    n137 = call <vilib>:"niFPGA Boolean Crossing.vi"("input"=w120, "direction"=w122) -> ("crossing"=w169:bool)  [unwired: 7 in]
    n138 = feedback #1() -> (w212:bool)
    n139 = Or(x=w120, y=w212) -> (x .or. y?=w154:bool)
    n140 = call "All Breaker Error Delay.vi"("Delay (Ticks)"="All Breaker Tick Limit", "Reset"=w126, "All Breakers Closed"=w129) -> ("All Breaker Err Out"=w127:bool)  [unwired: 7 in, 1 out]
    "All Breakers Fault" <- w127
    n141 = Build Array (concatenate)(w208, w152, w207, w173, w206, w184, w182, w181, w180, w179, w178, w149, w139, w148, w127) -> (w205:bool[])
    n142 = Boolean Array To Number(Boolean array=w205) -> (number=w200:u64)
    n143 = case shown="True" w126 {
      frame False {
      }
      frame True {
        n144 = local write "DAQ Zero Fault"(FALSE ("Reset Breaker")) -> ()
      }
    }
    n145 = feedback #2() -> (w135:bool)
    n146 = Not(x=w135) -> (.not. x?=w151:bool)
    n147 = Or(x=w135, y=w126) -> (x .or. y?=w172:bool)
    n148 = Compound Arithmetic op=OR(w127, w148, w139, w149, invert w121, w152, w216, w215, w174, w214, invert w172) -> (invert w137:bool)
    n149 = Build Array (concatenate)(w144, w143, w193, w142, w141, w196, w175, w158, w159, w160, w155, w161, w162, w153, w150, w151, w147, w146, w117) -> (w197:bool[])
    n150 = Compound Arithmetic op=OR(w117, w146, w147, w151, w150, w162, w161, w155, w160, w159, w158, w211, w176, invert w154, invert w121) -> (invert w210:bool)
    "PS Enable" <- w210
    n151 = feedback-in #1(w210) -> ()
    n152 = call "Breaker Enable Logic.vi"("Breaker Enable In"=w135, "Reset"=w126, "Fault OK"=w137, "Breaker Error"=w200) -> ("Resetting"=w170:bool, "Breaker First Error"=→"Breaker First Error":u64, "Breaker Enable Out"=w136:bool)  [unwired: 5 in]
    "Breaker Enable" <- w136
    n153 = Boolean Array To Number(Boolean array=w197) -> (number=w190:u32)
    n154 = xnode "FPGA I/O Node"("PS Enable Out"=w210) -> ()  [unwired: 1 in, 1 out]
    n155 = call <vilib>:"niFPGA Boolean Crossing.vi"("input"=w210, "direction"=enum8{"either", "false-true", "true-false"}."true-false") -> ("crossing"=w198:bool)  [unwired: 7 in]
    n156 = case shown="True" w170 {
      frame False {
      }
      frame True {
        n157 = local write "DAQ Zero Fault Channel"(bool[] [FALSE, FALSE, FALSE, FALSE, FALSE, FALSE, FALSE, FALSE, FALSE, FALSE, FALSE, FALSE, FALSE, FALSE, FALSE, FALSE, FALSE, FALSE, FALSE, FALSE, FALSE, FALSE, FALSE, FALSE, FALSE, FALSE, FALSE, FALSE, FALSE, FALSE, FALSE, FALSE, FALSE, FALSE, FALSE, FALSE, FALSE, FALSE] ("DAQ Fault Channel")) -> ()
      }
    }
    n158 = feedback-in #2(w136) -> ()
    n159 = feedback #3(u32 0 ("t")) -> (w187:u32)
    n160 = Select(t=u32 0, s=w169, f=w187) -> (s? t:f=w186:u32)
    n161 = local read "stop"() -> (w217:bool)
    n162 = Select(t=w190, s=w198, f=w186) -> (s? t:f=w189:u32)
    "PS Enable First Error" <- w189
    n163 = feedback-in #3(w189) -> ()
    n164 = case shown="True" w169 {
      frame False {
      }
      frame True {
        n165 = local write "Reset PS Enable"(FALSE ("Reset PS Enable")) -> ()
      }
    }
    n166 = xnode "FPGA I/O Node"("Breaker Enable Out"=w136) -> ()  [unwired: 1 in, 1 out]
    "PS Enable Loop WDT" <- TRUE
    "PS Enable Index" <- w177
  }
  n167 = while {
    tunnel: w2 -> [w226]
    i -> [w224]
    stop <- w225 stop-if-true
    # "Calibrate Loop"
    n168 = call "Loop Timer3"("Count(uSec)"=u32 100) -> ()  [unwired: 1 out]
    n169 = case shown="\"Zero Voltage\", \"Calibrate Voltage\"" "Input Select" {
      selector: "Input Select" -> [_ w230]
      tunnel: w226 -> [_ w229]
      frame "Input Voltage", Default {
      }
      frame "Zero Voltage", "Calibrate Voltage" {
        n170 = local read "Low Current Mode"() -> (w228:bool)
        n171 = case shown="True" w228 {
          tunnel: w230 -> [_ w241]
          tunnel: w229 -> [_ w236]
          frame False {
            n172 = local write "Input Select"(T1."Input Voltage" ("Input Select")) -> ()
          }
          frame True {
            n173 = flat-sequence {
              tunnel: w236 -> [w244]
              tunnel: [w243] -> w242
              tunnel: w235 -> [w246]
              tunnel: w242 -> [w247]
              tunnel: [w247] -> w234
              tunnel: [w246] -> w232
              frame #0 {
                n174 = xnode "FPGA I/O Node"("I/O Item"=TRUE ("Connector0/DIO0"), "FPGA I/O In"=w244) -> ("FPGA I/O Out"=w243:refnum<k21>)
              }
              frame #1 {
                n175 = call "Wait5"("Count(uSec)"=w246) -> ()  [unwired: 1 out]
              }
            }
            n176 = Equal?(x=w241, y=T1."Zero Voltage") -> (x = y?=w239:bool)
            n177 = Select(t=u16 5000 ("Count(uSec)"), s=w239, f=u16 2500 ("Count(uSec)")) -> (s? t:f=w235:u16)
            n178 = call "Wait6"("Count(uSec)"=w232) -> ()  [unwired: 1 out]
            n179 = xnode "FPGA I/O Node"("I/O Item"=FALSE ("Connector0/DIO0"), "FPGA I/O In"=w234) -> ()  [unwired: 1 out]
          }
        }
      }
    }
    n180 = local read "stop"() -> (w225:bool)
    "Calibrate Loop Index" <- w224
  }
  n181 = while {
    tunnel: w3 -> [w295]
    i -> [w281]
    stop <- "stop" stop-if-true
    # "Digitize Loop"
    n182 = local read "Convert Clock Ticks"() -> (w257:u32)
    n183 = local read "Magnet Configuration Data"() -> (w292:T21)
    n184 = call "Tick Count7"() -> ("Tick Count(uSec)"=w288:u32)
    n185 = call "Wait9"("Count(Ticks)"=w257) -> ("Tick Count(Ticks)"=w296:u32)
    n186 = feedback #4(u32 0 ("Tick Count(uSec)")) -> (w289:u32)
    n187 = Subtract(x=w288, y=w289) -> (x-y=→"uSec/Cycle":u32)
    n188 = feedback-in #4(w288) -> ()
    n189 = flat-sequence {
      tunnel: w296 -> [_]
      tunnel: w295 -> [w300]
      tunnel: [w299] -> w294
      frame #0 {
        n190 = xnode "FPGA I/O Node"("I/O Item"=TRUE ("Connector0/DIO0"), "FPGA I/O In"=w300) -> ("FPGA I/O Out"=w299:refnum<k21>)
      }
    }
    n191 = Unbundle By Name(w292) -> ("Scale Factors"=w256:T8[])
    n192 = Select(t=Digitizer_State_Enum."Reset", s="Reset Digitizers", f=Digitizer_State_Enum."StartCnvt" ("t")) -> (s? t:f=w297:T27)
    n193 = case shown="\"StartCnvt\"" w297 {
      tunnel: w294 -> [w308 w330]
      tunnel: [T28 [0.0, 0.0, 0.0, 0.0, 0.0, 0.0, 0.0, 0.0, 0.0, 0.0, 0.0, 0.0, 0.0, 0.0, 0.0, 0.0, 0.0, 0.0, 0.0, 0.0, 0.0, 0.0, 0.0, 0.0, 0.0, 0.0, 0.0, 0.0, 0.0, 0.0, 0.0, 0.0, 0.0, 0.0, 0.0, 0.0, 0.0, 0.0, 0.0, 0.0, 0.0, 0.0, 0.0, 0.0, 0.0, 0.0, 0.0, 0.0, 0.0, 0.0, 0.0, 0.0, 0.0, 0.0] ("Array") w328] -> w290
      tunnel: "Reset Digitizers" -> [w304 _]
      frame "Reset", Default {
        n194 = flat-sequence {
          tunnel: [w312] -> w309
          tunnel: w308 -> [w312]
          tunnel: "Digitize Reset Ticks" -> [w311]
          frame #0 {
            # "Delay for Digitzer Reset"
            n195 = call "Wait3"("Count(Ticks)"=w311) -> ()  [unwired: 1 out]
          }
        }
        n196 = call "Timer No Reset.vi"("Direction"=enum8{"either", "false-true", "true-false"}."false-true", "Tick Count(Ticks)"="Reset Digitizer Ticks", "Start Timer"=w304) -> ("Timer Running"=w302:bool)  [unwired: 8 in]
        n197 = local write "Reset Digitizers"(w302) -> ()
        n198 = xnode "FPGA I/O Node"("I/O Item"=FALSE ("Connector0/DIO0"), "FPGA I/O In"=w309) -> ()  [unwired: 1 out]
      }
      frame "StartCnvt" {
        n199 = flat-sequence {
          tunnel: [w401] -> w329
          tunnel: w330 -> [w401]
          tunnel: "Digitize Convert Ticks" -> [w400]
          frame #0 {
            # "Convert"
            n200 = call "Wait4"("Count(Ticks)"=w400) -> ()  [unwired: 1 out]
          }
        }
        n201 = local read "Input Select"() -> (w325:T1)
        n202 = call "Digitizer Clock In Data.vi"("Digitize Read Delay Ticks"="Digitize Read Delay Ticks", "Digitize # Bits"="Digitize # Bits", "Convert Clock Ticks"="Convert Clock Ticks", "Refnum in"=w329) -> ("Data Out"=w314:T23)  [unwired: 7 in]
        n203 = local read "Offset"() -> (w326:T23)
        n204 = case shown="\"Zero Voltage\"" w325 {
          tunnel: w314 -> [w347 w349 w375]
          tunnel: [w347 w348 w376] -> w313
          frame "Input Voltage", Default {
            n205 = xnode ("Memory Method Node")("Address"=u32 0, "Data"=w347) -> ()  [unwired: 1 in, 1 out]
          }
          frame "Zero Voltage" {
            n206 = disable-structure shown="Default" {
              disable-tunnel: w349 -> [w359 _]
              disable-tunnel: [w359 w360] -> w350
              frame condition #0 (active) {
              }
              frame condition #1 {
                n207 = Initialize Array(i16 1 ("Numeric"), 38 ("dimension size")) -> (w360:i16[])
              }
            }
            n208 = local read "Calibrate Index"() -> (w357:i16)
            n209 = Increment(x=w357) -> (x+1=w351:i16)
            "Calibrate Index" <- w351
            n210 = call "Dither Last Raw Data Value.vi"() -> ("Data"=w348:i16[])  [unwired: 11 in]
            n211 = Greater?(x=w351, y=i16 512) -> (0:w356:bool)
            n212 = Greater?(x=w351, y=i16 1536) -> (0:w354:bool)
            n213 = feedback #5() -> (w352:i32[])  [unwired: 1 in]
            n214 = case shown="True" w356 {
              tunnel: w350 -> [_ w373]
              tunnel: [T23 [0, 0, 0, 0, 0, 0, 0, 0, 0, 0, 0, 0, 0, 0, 0, 0, 0, 0, 0, 0, 0, 0, 0, 0, 0, 0, 0, 0, 0, 0, 0, 0, 0, 0, 0, 0, 0, 0] ("Scale") w372] -> w353
              tunnel: w352 -> [_ w371]
              frame False {
              }
              frame True {
                n215 = Add(x=w373, y=w371) -> (x+y=w372:i32[])
              }
            }
            n216 = feedback-in #5(w353) -> ()
            n217 = case shown="True" w354 {
              tunnel: w353 -> [_ w368]
              frame False {
              }
              frame True {
                n218 = Add(x=w368, y=512 ("n")) -> (x+y=w364:i32[])
                n219 = local write "Calibrate Index"(i16 0 ("Calibrate Index")) -> ()
                n220 = Scale By Power Of 2(n=i16 -10, x=w364) -> (x*2^n=→"Offset":i32[])
                n221 = local write "Input Select"(T1."Calibrate Voltage" ("Input Select")) -> ()
              }
            }
          }
          frame "Calibrate Voltage" {
            n222 = disable-structure shown="Default" {
              disable-tunnel: w375 -> [w385 _]
              disable-tunnel: [w385 w386] -> w374
              frame condition #0 (active) {
              }
              frame condition #1 {
                n223 = Initialize Array(29491 ("Numeric"), 38 ("dimension size")) -> (w386:i32[])
              }
            }
            n224 = local read "Calibrate Index"() -> (w383:i16)
            n225 = Increment(x=w383) -> (x+1=w377:i16)
            n226 = local write "Calibrate Index"(w377) -> ()
            n227 = call "Dither Last Raw Data Value.vi"() -> ("Data"=w376:i16[])  [unwired: 11 in]
            n228 = Greater?(x=w377, y=i16 512) -> (0:w382:bool)
            n229 = Greater?(x=w377, y=i16 1536) -> (0:w380:bool)
            n230 = feedback #6() -> (w378:i32[])  [unwired: 1 in]
            n231 = case shown="True" w382 {
              tunnel: w374 -> [_ w399]
              tunnel: [T23 [0, 0, 0, 0, 0, 0, 0, 0, 0, 0, 0, 0, 0, 0, 0, 0, 0, 0, 0, 0, 0, 0, 0, 0, 0, 0, 0, 0, 0, 0, 0, 0, 0, 0, 0, 0, 0, 0] ("Scale") w398] -> w379
              tunnel: w378 -> [_ w397]
              frame False {
              }
              frame True {
                n232 = Add(x=w399, y=w397) -> (x+y=w398:i32[])
              }
            }
            n233 = feedback-in #6(w379) -> ()
            n234 = case shown="True" w380 {
              tunnel: w379 -> [_ w394]
              frame False {
              }
              frame True {
                n235 = Add(x=w394, y=512 ("n")) -> (x+y=w390:i32[])
                n236 = local write "Calibrate Index"(i16 0 ("Calibrate Index")) -> ()
                n237 = Scale By Power Of 2(n=i16 -10, x=w390) -> (x*2^n=→"Scale":i32[])
                n238 = local write "Input Select"(T1."Input Voltage" ("Input Select")) -> ()
              }
            }
          }
        }
        "16 Bigitizer output" <- w313
        n239 = call "Check Digitizer Zeros.vi"("# Consecutive Zeros Fault"="# Consecutive Zeros Fault", "DAQ Raw Data"=w313) -> ("DAQ Zero Fault"=w320:bool, "DAQ Zero Fault Channel"=w322:bool[])  [unwired: 8 in]
        n240 = Subtract(x=w313, y=w326) -> (x-y=w324:fxp<+/-,17,17>[])
        n241 = call "Add ResMag Analog Channels FXP.vi"("Array in"=w324) -> ("Array out"=w327:T29)  [unwired: 10 in]
        n242 = case shown="True" w320 {
          selector: w320 -> [_ w344]
          tunnel: w322 -> [_ w345]
          frame False {
          }
          frame True {
            "DAQ Zero Fault Channel" <- w345
            "DAQ Zero Fault" <- w344
          }
        }
        n243 = call "Add Pressure Channels.vi"("Array in"=w327) -> ("Array Out"=w323:T28)  [unwired: 10 in]
        n244 = case shown="True" "Signal Injection On" {
          tunnel: [w331 w332] -> w328
          tunnel: w323 -> [w331 w336]
          frame False {
          }
          frame True {
            n245 = Divide(x="Inject frequency (Hz)", y=fxp<+,32,26> 40000000.0) -> (x/y=w341:fxp<+,64,22>)
            n246 = To Fixed-Point(fixed-point type=fxp<+,32,0> 0.0 ("frequency (periods/tick)"), number=w341) -> (fixed-point=w339:fxp<+,32,0>)
            n247 = call "Sine Wave Generator"("frequency (periods/tick)"=w339) -> ("sine out"=w343:i16)  [unwired: 14 in]
            n248 = xnode "Reinterpret Number"("x"=w343) -> ("y"=w335:fxp<+/-,16,5>)
            n249 = Add(x=w335, y="Inject Offset") -> (x+y=w334:fxp<+/-,19,5>)
            n250 = Replace Array Subset(array=w336, new element=w334, index="Inject Channel") -> (w332:T28)
          }
        }
      }
    }
    n251 = call "Loop Timer"("Count(Ticks)"="DAQ Cycle Ticks") -> ()  [unwired: 1 out]
    n252 = Index Array(array=w256, index=6) -> (element=w259:T8)
    n253 = Build Array (concatenate)(w256, w259) -> (w260:T8[])
    n254 = Build Array (concatenate)("Layer Scale Factors", "Co-Wound Scale Factor", "Dump Resistor Scale Factor", "Joint Scale Factors", "SC Bus Scale", w260, "Pressure Scale Factor") -> (w282:T8[])
    n255 = feedback-in #7(w290) -> ()
    n256 = feedback #7() -> (w271:T28)  [unwired: 1 in]
    n257 = Multiply(x=w282, y=w271) -> (x*y=w258:T8[])
    "Raw Data" <- w258
    n258 = call "Write UnFiltered FIFO 2 RT with Sync Guard.vi"("Sync Guard Data"="Sync Guard Data", "Raw Array Out"=w258) -> ("Timeout"=→"Timed Out? FIFO2RT Raw":bool)  [unwired: 9 in]
    n259 = call "Sliding Average.vi"("Ln2 Filter Size"="Ln2 Filter Size", "Array In"=w258) -> ("Filtered Array Out"=w275:T26)  [unwired: 9 in]
    "Filt Data" <- w275
    n260 = call "Write Filtered FIFO 2 RT with Sync Guard.vi"("Sync Guard Data"="Sync Guard Data", "Filtered Array Data"=w275) -> ("Timeout"=→"Timed Out? FIFO2RT Filter":bool)  [unwired: 9 in]
    n261 = call "Write Internal FPGA FIFOs.vi"("Filtered Array In"=w275) -> ("Timout"=w264:bool, "Dump Resistor Voltage"=→"Dump Resistor Voltage":T8)  [unwired: 9 in]
    n262 = Array Size(array=w275) -> (size(s)=→"Data Size":i32)
    n263 = Array Subset(array=w258, index=50, length=4) -> (w274:T8[])
    n264 = xnode ("FIFO Method Node")("Element"=w274, "Timeout"=4) -> ("Timed Out?"=w249:bool)  [unwired: 1 in, 1 out]
    n265 = local read "Reset Digitizers"() -> (w266:bool)
    n266 = Not(x=w266) -> (.not. x?=w265:bool)
    n267 = Or(x=w264, y=w249) -> (x .or. y?=w250:bool)
    n268 = feedback #8(FALSE) -> (w268:bool)
    n269 = And(x=w265, y=w268) -> (x .and. y?=w267:bool)
    n270 = Or(x=w250, y=w267) -> (x .or. y?=w263:bool)
    "Timed Out? FIFO Raw" <- w263
    n271 = feedback-in #8(w263) -> ()
    "Main Index" <- w281
    "DAQ Loop WDT" <- TRUE ("DAQ Loop WDT")
  }
  n272 = while {
    i -> [w404]
    stop <- w410 stop-if-true
    # "Reset Loop"
    n273 = local read "Reset Digitizers"() -> (w405:bool)
    n274 = xnode "FPGA I/O Node"() -> ("Digitizer Read Valid"=w409:bool)  [unwired: 1 in, 1 out]
    n275 = feedback #9(TRUE) -> (w407:bool)
    n276 = Or(x=w405, y=w407) -> (x .or. y?=w406:bool)
    n277 = And(x=w409, y=w406) -> (x .and. y?=w408:bool)
    "Digitizer Read OK" <- w408
    n278 = feedback-in #9(w408) -> ()
    n279 = call "Loop Timer4"("Count(uSec)"=u32 50) -> ()  [unwired: 1 out]
    n280 = local read "stop"() -> (w410:bool)
    "Read Error Index" <- w404
  }
  n281 = while {
    shift-right: [w416] -> _
    shift-left: w1 -> [w411]
    i -> [w412]
    stop <- w414 stop-if-true
    # "Watchdog Loop"
    n282 = flat-sequence {
      frame #0 {
        # "Check All Timers"
        n283 = local read "Co-Wound Loop WDT"() -> (w421:bool)
        "Co-Wound Loop WDT OK" <- w421
        n284 = local read "PS Enable Loop WDT"() -> (w420:bool)
        "PS Enable Loop WDT OK" <- w420
        n285 = local read "Resistive Loop WDT"() -> (→"Resistive Loop WDT OK":bool)
        n286 = local read "Pressure Loop WDT"() -> (→"Pressure Loop WDT OK":bool)
        n287 = local read "SC Bus Loop WDT"() -> (w423:bool)
        "SC Bus Loop WDT OK" <- w423
        n288 = local read "Layer Loop WDT"() -> (w426:bool)
        "Layer Loop WDT OK" <- w426
        n289 = local read "Joint Loop WDT"() -> (w424:bool)
        "Joint Loop WDT OK" <- w424
        n290 = local read "DAQ Loop WDT"() -> (w425:bool)
        "DAQ Loop WDT OK" <- w425
        n291 = Compound Arithmetic op=AND(w426, w425, w424, w421, w423, w420) -> (→"Overall WDT":bool)
        n292 = case shown="False" w420 {
          frame False {
            w428 = FALSE ("Calc Loop WDT")
            # "PS Enable Loop stopped!!"
            n293 = local write "Breaker Enable"(w428) -> ()
            n294 = local write "PS Enable"(w428) -> ()
            n295 = xnode "FPGA I/O Node"("Breaker Enable Out"=w428, "PS Enable Out"=w428) -> ()  [unwired: 2 in, 2 out]
          }
          frame True {
          }
        }
      }
      frame #1 {
        w429 = FALSE ("Calc Loop WDT")
        # "Reset All Timers"
        n296 = local write "SC Bus Loop WDT"(w429) -> ()
        n297 = local write "Layer Loop WDT"(w429) -> ()
        n298 = local write "Pressure Loop WDT"(w429) -> ()
        n299 = local write "Co-Wound Loop WDT"(w429) -> ()
        n300 = local write "Joint Loop WDT"(w429) -> ()
        n301 = local write "PS Enable Loop WDT"(w429) -> ()
        n302 = local write "Resistive Loop WDT"(w429) -> ()
        n303 = local write "DAQ Loop WDT"(w429) -> ()
      }
      frame #2 {
        w438 = T1."Input Voltage" ("Input Select")
        # "Wait Loop 0.05 Sec"
        n304 = xnode "FPGA I/O Node"() -> ("Chassis Temperature"=w452:i16, "Pwr +/-15V Pri Err"=→"Pwr ±15V Pri Err":bool, "Pwr +/-15V Aux Err"=→"Pwr ±15V Aux Err":bool, "Pwr 5V Pri Err"=→"Pwr 5V Pri Err":bool, "Pwr 5V Aux Err"=→"Pwr 5V Aux Err":bool, "Pwr 24V Pri Err"=→"Pwr 24V Pri Err":bool, "Pwr 24V Aux Err"=→"Pwr 24V Aux Err":bool, "Pwr 125V Err"=→"Pwr 125V Err":bool)  [unwired: 8 in, 8 out]
        n305 = disable-structure shown="Default" {
          disable-tunnel: [w459 "Breaker 1"] -> w435
          disable-tunnel: [w458 "Breaker 2"] -> w434
          disable-tunnel: [w457 "Breaker 3"] -> w433
          disable-tunnel: [w456 "Breaker 4"] -> w430
          disable-tunnel: [w455 "Breaker 5"] -> w431
          disable-tunnel: [w454 "Breaker 6"] -> w432
          frame condition #0 (active) {
            n306 = xnode "FPGA I/O Node"() -> ("Breaker Pos 1 Closed"=w459:bool, "Breaker Pos2 Closed"=w458:bool, "Breaker Pos3 Closed"=w457:bool, "Breaker Neg1 Closed"=w456:bool, "Breaker Neg2 Closed"=w455:bool, "Breaker Neg3 Closed"=w454:bool)  [unwired: 6 in, 6 out]
          }
          frame condition #1 {
          }
        }
        "Breaker Pos 1 Closed" <- w435
        "Breaker Pos 2 Closed" <- w434
        "Breaker Pos 3 Closed" <- w433
        "Breaker Neg 4 Closed" <- w430
        "Breaker Neg 5 Closed" <- w431
        "Breaker Neg 6 Closed" <- w432
        n307 = To Fixed-Point(number=w452) -> (fixed-point=w449:fxp<+/-,16,14>)  [unwired: 1 in]
        n308 = Scale By Power Of 2(n=i16 -2 ("Chassis Temperature"), x=w449) -> (x*2^n=→"Chassis Temperature":fxp<+/-,16,14>)
        n309 = Compound Arithmetic op=AND(w432, w431, w430, w433, w434, w435) -> (→"All Breakers Closed":bool)
        n310 = local read "Input Select"() -> (w439:T1)
        n311 = call "Loop Timer2"("Count(Ticks)"=u32 2000000) -> ()  [unwired: 1 out]
        n312 = Not Equal?(x=w439, y=w438) -> (x != y?=w437:bool)
        n313 = call "Error Time Check.vi"("Ticks Until Trigger"=u32 20000000, "Limit Exceeded"=w437) -> ("Limit Triggered"=w440:bool)  [unwired: 9 in]
        n314 = case shown="True" w440 {
          tunnel: w438 -> [_ w466]
          frame False {
          }
          frame True {
            n315 = local write "Input Select"(w466) -> ()
          }
        }
      }
    }
    n316 = Boolean To (0,1)(Boolean=w411) -> (0, 1=w415:i16)
    n317 = xnode "FPGA I/O Node"("USER FPGA LED"=w415) -> ()  [unwired: 1 in, 1 out]
    n318 = local read "stop"() -> (w417:bool)
    n319 = disable-structure shown="Default" {
      disable-tunnel: w411 -> [w418 _]
      frame condition #0 (active) {
        n320 = xnode "FPGA I/O Node"("Watchdog Timer Out"=w418) -> ()  [unwired: 1 in, 1 out]
      }
      frame condition #1 {
      }
    }
    n321 = Or(x=w417, y="Stop WD Loop") -> (x .or. y?=w414:bool)
    n322 = Not(x=w411) -> (.not. x?=w416:bool)
    "Watch Dog Index" <- w412
  }
  n323 = while {
    i -> [w476]
    stop <- w481 stop-if-true
    # "Co-Wound Check Loop"
    n324 = xnode ("FIFO Method Node")("Timeout"=-1) -> ("Element"=w478:fxp<+/-,38,12>[], "Timed Out?"=w480:bool)  [unwired: 1 in, 1 out]
    "Timed Out? Co-Wound Read" <- w480
    "CoWound Volt Array" <- w478
    n325 = local read "Low Current Mode"() -> (w471:bool)
    n326 = local read "Low Current Delay Factor"() -> (w470:u16)
    n327 = local read "stop"() -> (w482:bool)
    n328 = Increment(x="Co-Wound Asymmetry Factor") -> (x+1=w477:fxp<+,17,1>)
    n329 = Index Array(array=w478) -> (element #1=w486:fxp<+/-,38,12>, element #2=w488:fxp<+/-,38,12>)  [unwired: 2 in]
    n330 = Or(x=w482, y=w480) -> (x .or. y?=w481:bool)
    n331 = Multiply(x=w488, y=w477) -> (x*y=w487:fxp<+/-,54,12>)
    n332 = Subtract(x=w486, y=w487) -> (x-y=w485:fxp<+/-,38,12>)
    n333 = Select(t=w470, s=w471, f=u16 1) -> (s? t:f=w473:u16)
    n334 = Absolute Value(x=w485) -> (abs(x)=w484:fxp<+,38,12>)
    n335 = Greater?(x=w484, y="CoWound Volt Limit") -> (0:w475:bool)
    "Proto Co-Wournd Limit" <- w475
    n336 = Multiply(x=w473, y="CoWound Tick Limit") -> (x*y=w468:u32)
    n337 = call "Error Time Check.vi"("Ticks Until Trigger"=w468, "Limit Exceeded"=w475) -> ("Limit Triggered"=→"Co-Wound Limit Err":bool)  [unwired: 9 in]
    "Co-Wound Loop WDT" <- TRUE ("Co-Wound Loop WDT")
    "Co-Wound Index" <- w476
  }
  n338 = while {
    i -> [w499]
    stop <- w504 stop-if-true
    # "Joint Check Loop"
    n339 = xnode ("FIFO Method Node")("Timeout"=-1) -> ("Element"=w501:fxp<+/-,38,12>[], "Timed Out?"=w503:bool)  [unwired: 1 in, 1 out]
    "Timed Out? Joint Read" <- w503
    "Joint Voltages" <- w501
    n340 = local read "stop"() -> (w500:bool)
    n341 = Absolute Value(x=w501) -> (abs(x)=w507:fxp<+,38,12>[])
    n342 = local read "Low Current Mode"() -> (w494:bool)
    n343 = local read "Low Current Delay Factor"() -> (w493:u16)
    n344 = Greater?(x=w507, y="Joint Volt Limit") -> (0:w506:bool[])
    "Joint Err Array" <- w506
    n345 = Or(x=w503, y=w500) -> (x .or. y?=w504:bool)
    n346 = Or Array Elements(Boolean array=w506) -> (logical OR=w498:bool)
    "Proto Joint Volt" <- w498
    n347 = Select(t=w493, s=w494, f=u16 1) -> (s? t:f=w496:u16)
    n348 = Multiply(x=w496, y="Joint Tick Limit") -> (x*y=w491:u32)
    n349 = call "Error Time Check.vi"("Ticks Until Trigger"=w491, "Limit Exceeded"=w498) -> ("Limit Triggered"=→"Joint Limit Err":bool)  [unwired: 9 in]
    "Joint Loop WDT" <- TRUE ("Calc Loop WDT")
    "Joint Index" <- w499
  }
  n350 = while {
    i -> [w517]
    stop <- w520 stop-if-true
    w524 = 3 ("length")
    # "Pressure Check - Relief Valves"
    n351 = xnode ("FIFO Method Node")("Timeout"=-1) -> ("Element"=w525:fxp<+/-,38,12>[], "Timed Out?"=w519:bool)  [unwired: 1 in, 1 out]
    "Pressures" <- w525
    n352 = Select(t="Pressure Inlet Cooldown Limit", s="Cooldown Mode", f="Pressure Inlet Limit (BarA)") -> (s? t:f=w510:T24)
    n353 = Select(t="Pressure Outlet Cooldown Limit", s="Cooldown Mode", f="Pressure Outlet Limit (BarA)") -> (s? t:f=w512:T24)
    n354 = Index Array(array=w525, index=w524) -> (element=w523:fxp<+/-,38,12>)
    n355 = Array Subset(array=w525, length=w524) -> (w526:fxp<+/-,38,12>[])  [unwired: 1 in]
    n356 = Greater Or Equal?(x=w523, y=w512) -> (x >= y?=w518:bool)
    n357 = Greater?(x=w526, y=w510) -> (0:w529:bool[])
    n358 = local read "stop"() -> (w528:bool)
    n359 = Build Array (concatenate)(w529, w518) -> (w516:bool[])
    "Pressure Limit Err Array" <- w516
    n360 = Or Array Elements(Boolean array=w516) -> (logical OR=w521:bool)
    "Pressure Limit Err" <- w521
    n361 = Or(x=w519, y=w528) -> (x .or. y?=w520:bool)
    n362 = Not(x=w521) -> (.not. x?=w515:bool)
    n363 = call "Error Time Check.vi"("Ticks Until Trigger"="Ticks to Close Relief", "Limit Exceeded"=w515) -> ("Limit Triggered"=w514:bool)  [unwired: 9 in]
    n364 = xnode "FPGA I/O Node"("Pressure Relief Valve PIC751C"=w514) -> ()  [unwired: 1 in, 1 out]
    "Pressure Loop WDT" <- TRUE ("Pressure Loop WDT")
    "Pressure Check Index" <- w517
  }
  n365 = while {
    i -> [w544]
    stop <- w554 stop-if-true
    w555 = 16 ("x-y")
    # "Layer Voltage Tap Check Loop"
    n366 = xnode ("FIFO Method Node")("Timeout"=-1) -> ("Element"=w550:fxp<+/-,38,12>[], "Timed Out?"=w548:bool)  [unwired: 1 in, 1 out]
    "Layer Voltages" <- w550
    "Timed Out? Calc Read" <- w548
    n367 = local read "stop"() -> (w547:bool)
    n368 = Or(x=w548, y=w547) -> (x .or. y?=w554:bool)
    n369 = Array Subset(array=w550, index=1, length=w555) -> (w558:fxp<+/-,38,12>[])
    n370 = Array Subset(array=w550, index=0, length=w555) -> (w561:fxp<+/-,38,12>[])
    n371 = Array Subset(array=w550, index=2, length=w555) -> (w560:fxp<+/-,38,12>[])
    n372 = local read "Low Current Mode"() -> (w538:bool)
    n373 = Add(x=w561, y=w560) -> (x+y=w541:fxp<+/-,38,12>[])
    n374 = Increment(x="Fudge Factors") -> (x+1=w546:fxp<+/-,33,4>[])
    n375 = Scale By Power Of 2(n=i16 -1 ("y"), x=w541) -> (x*2^n=w542:fxp<+/-,38,12>[])
    n376 = Multiply(x=w546, y=w558) -> (x*y=w556:fxp<+/-,38,12>[])
    n377 = Subtract(x=w556, y=w542) -> (x-y=w552:fxp<+/-,38,12>[])
    "Error Voltages" <- w552
    n378 = Absolute Value(x=w552) -> (abs(x)=w553:fxp<+,38,12>[])
    n379 = Greater?(x=w553, y="VT Quench Volt Limit") -> (0:w545:bool[])
    "VT Error Array" <- w545
    n380 = Select(t="Low Current Delay Factor", s=w538, f=u16 1) -> (s? t:f=w536:u16)
    n381 = Or Array Elements(Boolean array=w545) -> (logical OR=w540:bool)
    "Proto VT Quench" <- w540
    n382 = Multiply(x=w536, y="VT Quench Tick Limit") -> (x*y=w533:u32)
    n383 = call "Error Time Check.vi"("Ticks Until Trigger"=w533, "Limit Exceeded"=w540) -> ("Limit Triggered"=→"VT Quench Err":bool)  [unwired: 9 in]
    "Layer Loop WDT" <- TRUE ("Calc Loop WDT")
    "Layer Index" <- w544
  }
  n384 = while {
    i -> [w608]
    stop <- w612 stop-if-true
    w577 = 6 ("length")
    w607 = 2 ("index")
    # "SC Bus Check Loop"
    n385 = xnode ("FIFO Method Node")("Timeout"=-1) -> ("Element"=w576:fxp<+/-,38,12>[], "Timed Out?"=w610:bool)  [unwired: 1 in, 1 out]
    "Timed Out? SC Bus Read" <- w610
    n386 = local read "stop"() -> (w613:bool)
    n387 = Or(x=w613, y=w610) -> (x .or. y?=w612:bool)
    n388 = Array Subset(array=w576, length=w577) -> (w578:fxp<+/-,38,12>[])  [unwired: 1 in]
    "SC Bus Volt Array" <- w578
    n389 = local read "Low Current Mode"() -> (w583:bool)
    n390 = local read "Low Current Delay Factor"() -> (w582:u16)
    n391 = Absolute Value(x=w578) -> (abs(x)=w604:fxp<+,38,12>[])
    n392 = Array Subset(array=w604, index=w607, length=w607) -> (w566:fxp<+,38,12>[])
    n393 = Array Subset(array=w604, index=0, length=w607) -> (w575:fxp<+,38,12>[])
    n394 = Array Subset(array=w604, index=4, length=w607) -> (w601:fxp<+,38,12>[])
    n395 = Index Array(array=w576, index=w577) -> (element=w574:fxp<+/-,38,12>)
    n396 = Absolute Value(x=w574) -> (abs(x)=w570:fxp<+,38,12>)
    n397 = Select(t=w582, s=w583, f=u16 1) -> (s? t:f=w585:u16)
    n398 = Multiply(x="HTS Resistance (nOhm)", y=w570) -> (x*y=w572:T8[])
    n399 = Multiply(x=w585, y="SC Bus Tick Limit") -> (x*y=w579:u32)
    n400 = Add(x="HTS Offset (microV)", y=w572) -> (x+y=w565:T8[])
    n401 = Multiply(x=T8 9.98377799987793e-07 ("Numeric"), y=w565) -> (x*y=w571:T8[])
    n402 = Greater?(x=w601, y="SC Bus Limit") -> (0:w596:bool[])
    "SC Bus Err Array" <- w596
    n403 = Subtract(x=w566, y=w571) -> (x-y=w569:T8[])
    n404 = Absolute Value(x=w569) -> (abs(x)=w567:fxp<+,38,12>[])
    n405 = Greater?(x=w575, y="Res Lead Limit") -> (0:w595:bool[])
    "RT Bus Err Array" <- w595
    n406 = Greater?(x=w567, y="HTS Lead Warn") -> (0:→"HTS Lead Warn Err Array":bool[])
    n407 = Greater?(x=w567, y="HTS Lead FRZ") -> (0:→"HTS Lead FRZ Err Array":bool[])
    n408 = Greater?(x=w567, y="HTS Lead Trip") -> (0:w594:bool[])
    "HTS Bus Err Array" <- w594
    n409 = Or Array Elements(Boolean array=w596) -> (logical OR=w593:bool)
    "Proto SC Bus Limit" <- w593
    n410 = Or Array Elements(Boolean array=w594) -> (logical OR=w592:bool)
    "Proto HTS Bus Limit" <- w592
    n411 = Or Array Elements(Boolean array=w595) -> (logical OR=w591:bool)
    "Proto RT Bus Limit" <- w591
    n412 = call "Error Time Check.vi"("Ticks Until Trigger"=w579, "Limit Exceeded"=w593) -> ("Limit Triggered"=→"SC Bus Limit Err":bool)  [unwired: 9 in]
    n413 = call "Error Time Check.vi"("Ticks Until Trigger"="HTS Lead Tick Limit", "Limit Exceeded"=w592) -> ("Limit Triggered"=→"HTS Bus Limit Err":bool)  [unwired: 9 in]
    n414 = call "Error Time Check.vi"("Ticks Until Trigger"="Res Lead Tick Limit", "Limit Exceeded"=w591) -> ("Limit Triggered"=→"RT Bus Limit Err":bool)  [unwired: 9 in]
    "SC Bus Loop WDT" <- TRUE ("SC Bus Loop WDT")
    "SC Bus Index" <- w608
  }
